vi "Main On Load Action VI.vi"(8 "error in (no error)":errorcluster, 11 "Device Item Ref in":T1 format="%.0x") -> (0 "error out":errorcluster, 3 "Device Item Ref out":T1 format="%.0x")   [LabVIEW 2011, in "Sensor Simulation Custom Device.lvlib"]
uses:
  Sensor Simulation Custom Device.lvlib
  <vilib>/NI Veristand/Custom Device API/Custom Device Item Ref.ctl
  <vilib>/NI Veristand/Custom Device API/Custom Device Execution Mode.ctl
  <vilib>/NI Veristand/Custom Device API/Custom Device Supported Target.ctl
  <vilib>/NI Veristand/Custom Device API/Path Type.ctl
  <vilib>/NI Veristand/Custom Device API/Custom Device Path Data.ctl
  <vilib>/NI Veristand/Custom Device API/Path Specification.ctl
  Global.vi
  <vilib>/NI Veristand/Custom Device API/Get Item Property (Dependent File).vi
  <vilib>/NI Veristand/Custom Device API/Set Item Property (Path).vi
  <vilib>/NI Veristand/Custom Device API/Custom Device API.lvlib
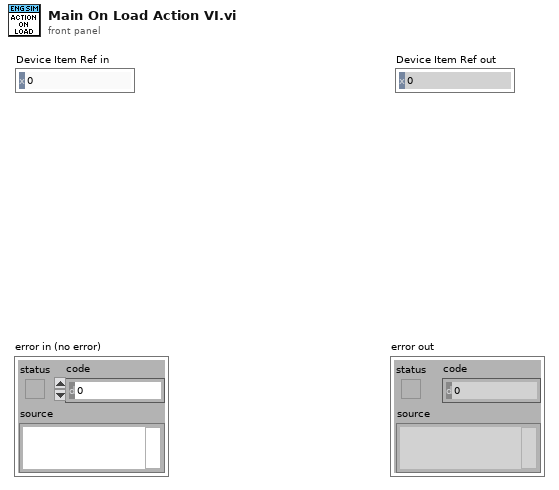
[diagram p1: front panel]
types:
  T1 = typedef "Custom Device API.lvlib/Custom Device Item Ref.ctl" = u64
  T2 = typedef "Custom Device API.lvlib/Custom Device Execution Mode.ctl" = enum16{"Asynchronous", "Inline HW Interface", "Inline Model Interface", "Inline Timing and Sync", "Asynchronous Timing and Sync"}
  T3 = typedef "Custom Device API.lvlib/Path Type.ctl" = enum16{"Absolute", "To Base", "To Common Data Dir", "To Application Data Dir"}
  T4 = typedef "Custom Device API.lvlib/Custom Device Supported Target.ctl" = enum16{"All", "PharLap", "VxWorks", "Windows", "PharLap & Windows", "PharLap & VxWorks", "VxWorks & Windows"}
  T5 = typedef "Custom Device API.lvlib/Dependent File Optional Info.ctl" = cluster{"Version":string, "RTDestination":path, "ForceDownload":bool, "SupportedTarget":string, "MD5":string}
  T6 = typedef "Custom Device API.lvlib/Custom Device Path Data.ctl" = cluster{"SupportedTarget":T4, "Source":T7, "RT Destination":path}
  T7 = typedef "Custom Device API.lvlib/Path Specification.ctl" = cluster{"Path":path, "Type":T3}
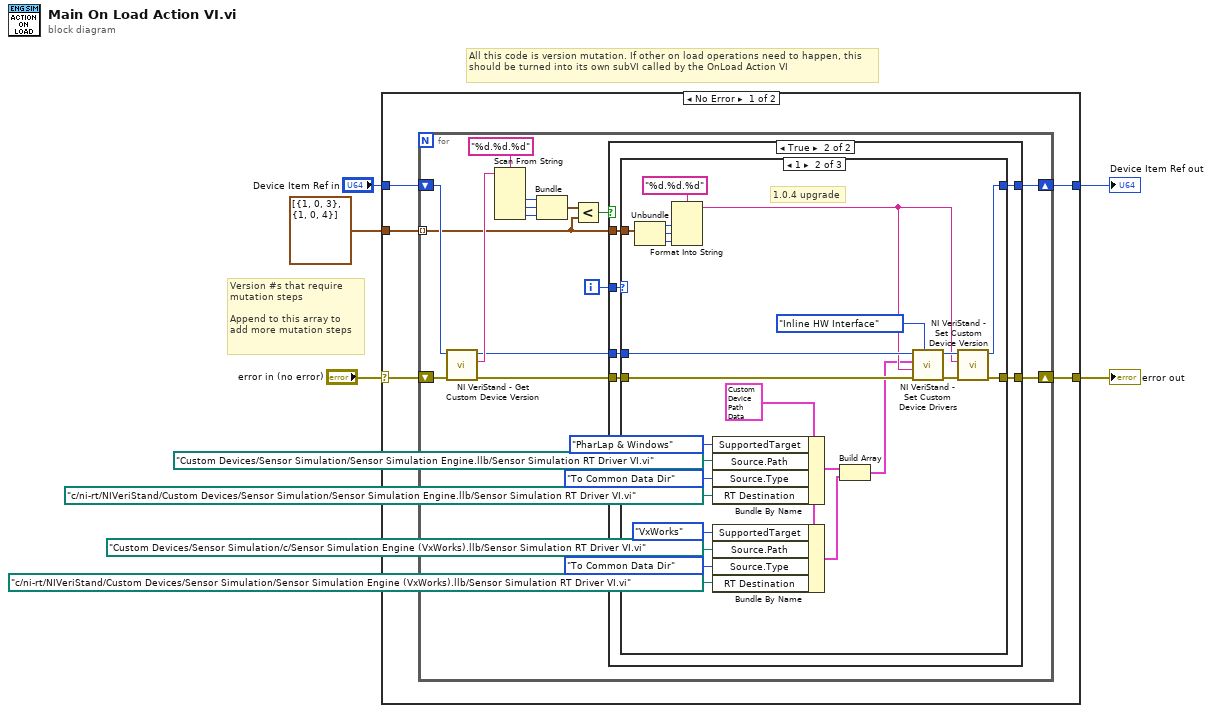
[diagram p0: block diagram]
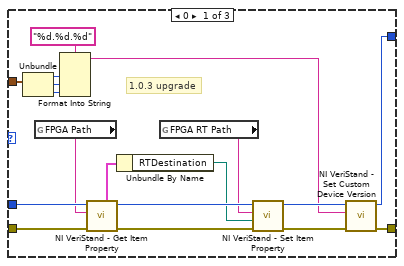
[diagram p3: hidden frame]
diagram:
  # "All this code is version mutation. If other on load operations need to happen, this should be turned into its own subVI called by the OnLoad Action VI"
  # "Version #s that require\nmutation steps\n\nAppend to this array to\nadd more mutation steps"
  n1 = case shown="No Error" "error in (no error)" {
    selector: "error in (no error)" -> [w9 w80]
    tunnel: [w6 w80] -> w4
    tunnel: "Device Item Ref in" -> [w8 w79]
    tunnel: [w7 w79] -> w2
    tunnel: cluster{i32, i32, i32}[] [{1, 0, 3}, {1, 0, 4}] -> [w10 _]
    frame No Error {
      n2 = for {
        tunnel: w10 -> [w12] mode=indexing
        shift-right: [w16] -> w6
        shift-left: w9 -> [w21]
        shift-right: [w14] -> w7
        shift-left: w8 -> [w20]
        i -> [w13]
        n3 = call <vilib>:"NI VeriStand - Get Custom Device Version.vi"("error in (no error)"=w21, "Device Ref in"=w20) -> ("error out"=w17:errorcluster, "Value"=w19:string, "Device Ref out"=w15:T1)  [unwired: 7 in]
        n4 = Scan From String(format string="%d.%d.%d", input string=w19) -> (output 1=w23:i32, output 2=w24:i32, output 3=w11:i32)  [unwired: 5 in, 3 out]
        n5 = Bundle(w23, w24, w11) -> (w25:cluster{i32, i32, i32})  [unwired: 1 in]
        n6 = Less?(x=w25, y=w12) -> (x < y?=w18:bool)
        n7 = case shown="True" w18 {
          tunnel: w17 -> [w27 w33]
          tunnel: [w27 w32] -> w16
          tunnel: w15 -> [w26 w29]
          tunnel: [w26 w30] -> w14
          tunnel: w13 -> [_ w31]
          tunnel: w12 -> [_ w28]
          frame False {
          }
          frame True {
            n8 = case shown="1" w31 {
              tunnel: w33 -> [w50 w75 w78]
              tunnel: [w51 w76 w78] -> w32
              tunnel: [w37 w70 w77] -> w30
              tunnel: w29 -> [w49 w67 w77]
              tunnel: w28 -> [w39 w71 _]
              frame 0 {
                # "1.0.3 upgrade"
                n9 = Unbundle(w39) -> (w41:i32, w42:i32, w36:i32)
                n10 = global read "Global.vi" "FPGA Path"() -> (w35:string)
                n11 = Format Into String(format string="%d.%d.%d", w41, w42, w36) -> (resulting string=w38:string)  [unwired: 2 in, 1 out]
                n12 = call-poly <vilib>:"NI VeriStand - Get Item Property.vi"("error in (no error)"=w50, "Property Name"=w35, "Item Ref in"=w49) -> ("error out"=w47:errorcluster, "Item Ref out"=w46:T1, "OptionalInfo"=w48:T5)  [unwired: 4 in, 2 out]
                n13 = Unbundle By Name(w48) -> ("RTDestination"=w45:path)
                n14 = global read "Global.vi" "FPGA RT Path"() -> (w34:string)
                n15 = call-poly <vilib>:"NI VeriStand - Set Item Property.vi"("error in (no error)"=w47, "Value"=w45, "Property Name"=w34, "Item Ref in"=w46) -> ("error out"=w44:errorcluster, "Item Ref out"=w43:T1)  [unwired: 5 in, 1 out]
                n16 = call <vilib>:"NI VeriStand - Set Custom Device Version.vi"("error in (no error)"=w44, "Value"=w38, "Device Ref in"=w43) -> ("error out"=w51:errorcluster, "Device Ref out"=w37:T1)  [unwired: 7 in]
              }
              frame 1 {
                w64 = T6 {"SupportedTarget"=enum."All", "Source"={"Path"=path "", "Type"=enum."Absolute"}, "RT Destination"=path ""} ("Driver VI Path")
                # "1.0.4 upgrade"
                n17 = Unbundle(w71) -> (w73:i32, w74:i32, w69:i32)
                n18 = Format Into String(format string="%d.%d.%d", w73, w74, w69) -> (resulting string=w65:string)  [unwired: 2 in, 1 out]
                n19 = Bundle By Name(cluster=w64, "SupportedTarget"=Custom_Device_Supported_Target."PharLap & Windows", "Source.Path"=path "Custom Devices/Sensor Simulation/Sensor Simulation Engine.llb/Sensor Simulation RT Driver VI.vi", "Source.Type"=Path_Type."To Common Data Dir", "RT Destination"=path "c:/ni-rt/NIVeriStand/Custom Devices/Sensor Simulation/Sensor Simulation Engine.llb/Sensor Simulation RT Driver VI.vi") -> (w63:T6)
                n20 = Bundle By Name(cluster=w64, "SupportedTarget"=Custom_Device_Supported_Target."VxWorks", "Source.Path"=path "Custom Devices/Sensor Simulation/c/Sensor Simulation Engine (VxWorks).llb/Sensor Simulation RT Driver VI.vi", "Source.Type"=Path_Type."To Common Data Dir", "RT Destination"=path "c:/ni-rt/NIVeriStand/Custom Devices/Sensor Simulation/Sensor Simulation Engine (VxWorks).llb/Sensor Simulation RT Driver VI.vi") -> (w62:T6)
                n21 = Build Array(w63, w62) -> (w61:T6[])
                n22 = call <vilib>:"NI VeriStand - Set Custom Device Drivers.vi"("Execution mode"=Custom_Device_Execution_Mode."Inline HW Interface", "error in (no error)"=w75, "Version"=w65, "Driver VI"=w61, "Device Ref in"=w67) -> ("error out"=w68:errorcluster, "Device Ref out"=w66:T1)  [unwired: 5 in]
                n23 = call <vilib>:"NI VeriStand - Set Custom Device Version.vi"("error in (no error)"=w68, "Value"=w65, "Device Ref in"=w66) -> ("error out"=w76:errorcluster, "Device Ref out"=w70:T1)  [unwired: 7 in]
              }
              frame Default {
              }
            }
          }
        }
      }
    }
    frame Error {
    }
  }
  "error out" <- w4
  "Device Item Ref out" <- w2
